vi "Global textParse.vi"() -> ()   [LabVIEW 2018]
panel:
  in  "Sense Voltage Tol. Max":string
  in  "Sense Voltage Tol. Min":string
  in  "Sense Voltage":string
  in  "Current Limit(@45% PWM)":string
  in  "Current Running Tol. Max":string
  in  "Current Running Tol. Min":string
  in  "Ircomp(@70% PWM)":string
  in  "Speed Pot Voltage Tol. Max":string
  in  "Speed Pot Voltage Tol. Min":string
  in  "Speed Pot Voltage High(@85% PWM)":string
  in  "Rated Output Current Tol. Max":string
  in  "Speed Pot Voltage Mid(@85% PWM)":string
  in  "Speed Pot Voltage Low(@85% PWM)":string
  in  "Voltage FET Driver Tol. Max":string
  in  "Voltage Micro Tol. Min":string
  out "Voltage Output Tol. Min":string
  out "Allowable Power Interuption":string
  out "Input Voltage Tol. Min":string
  out "Input Voltage Tol. Max":string
  in  "HV Bus Tol. Max":string
  in  "HV Bus Tol. Min":string
  in  "HV Bus Voltage(@10% PWM)":string
  in  "LED Frequency Max":string
  in  "LED Frequency Min":string
  in  "LED Frequency (Foldback)":string
  in  "LED Frequency (Limit)":string
  in  "LED Frequency (Charge)":string
  in  "Voltage FET Driver Tol. Min":string
  in  "Voltage FET Driver":string
  in  "Voltage Micro Tol. Max":string
  in  "Voltage Micro":string
  in  "Rated Output Current Tol. Min":string
  in  "Rated Output Current":string
  in  "Ripple/Noise Tol. Max":string
  in  "Ripple/Noise Tol. Min":string
  in  "Ripple/Noise":string
  in  "Voltage Output Tol. Max":string
  in  "Voltage Output":string
  in  "Max Input Current":string
  in  "Input Current":string
  in  "Input Voltage":string
  in  "Vendor Number":string
  in  "Vendor Name":string
  in  "Firmware":string
  in  "Part Number":string
  in  "Part Name":string
  # "Document data (0-4)"
  # "Input Primary  (7-11)"
  # "Output Secondary (14-21)"
  # "Output Primary (24-27)"
  # "Motor Controller (30-40)"
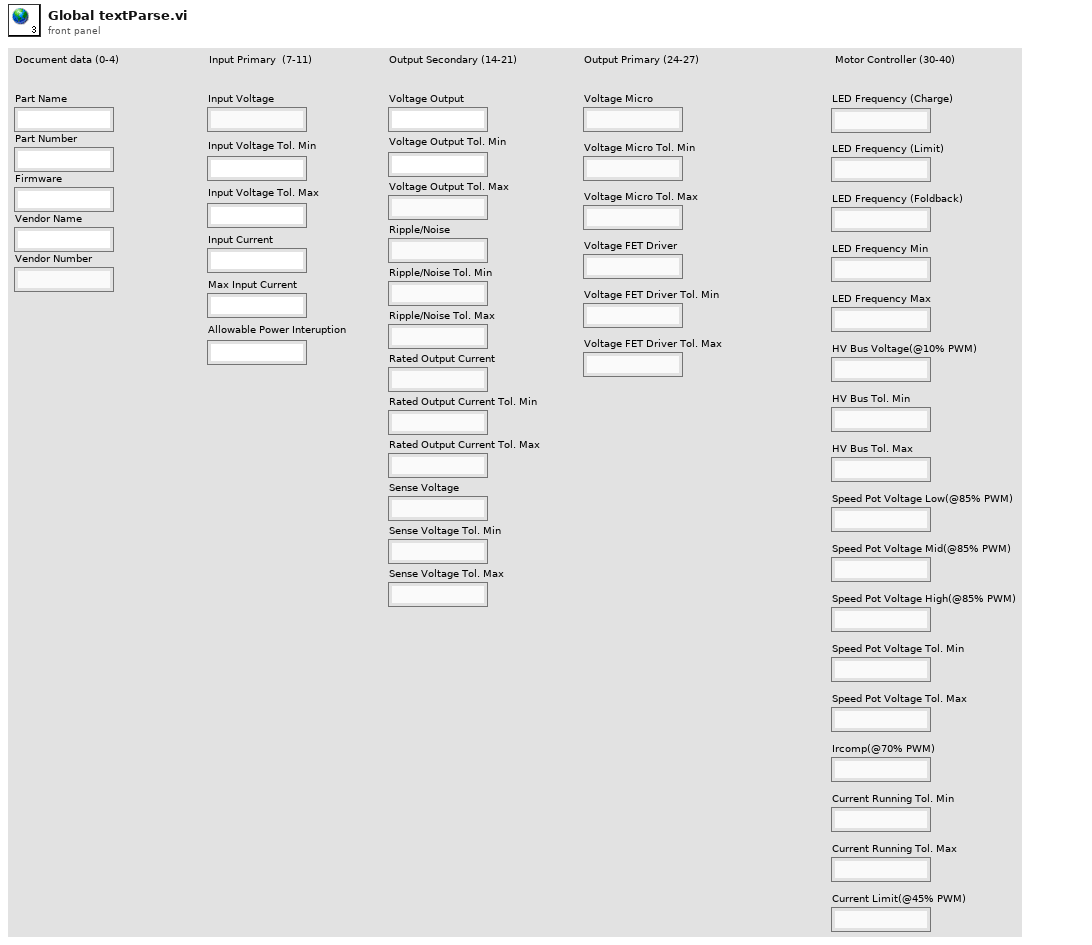
[diagram p1: front panel]
diagram:
